vi "Read.vi"(8 "error in (no error)":errorcluster) -> (0 "error out":errorcluster)   [LabVIEW 2018, in "text_file.lvlib"]
doc: "Reads all text (all contents) of file."
uses:
  text_file.lvlib
  private_data (library_variable).vi
panel:
  out "Text read from file (contents of file)":string
  # "Development\ncontrols/indicators useful for development and testing, but which are not outputs of the VI"
  # "Input\nInputs to the VI"
  # "Output\nOutputs of the VI"
  # "Description\n\nBlank VI with error handling case. \n\nSummarize the use of this VI in this space."
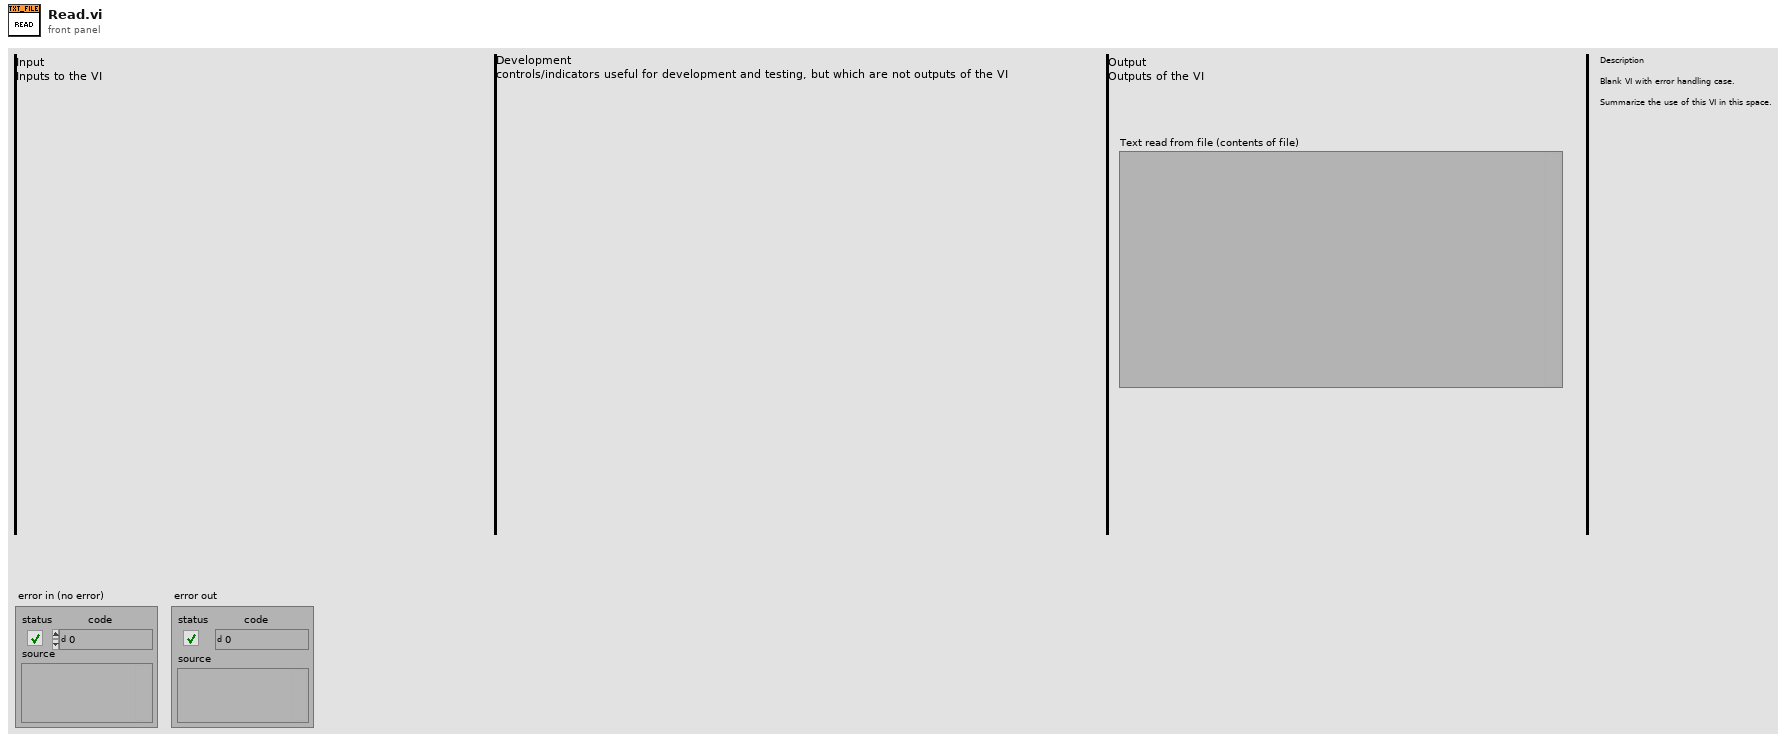
[diagram p1: front panel]
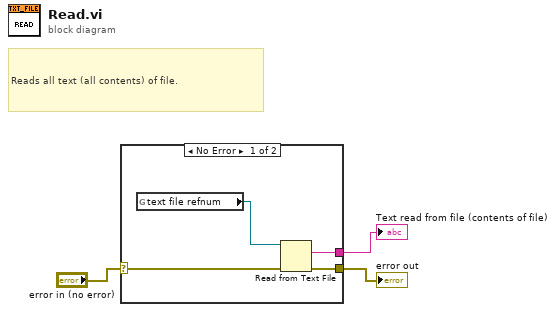
[diagram p0: block diagram]
diagram:
  # "Reads all text (all contents) of file."
  n1 = case shown="No Error" "error in (no error)" {
    selector: "error in (no error)" -> [w7 w8]
    tunnel: [w6 w8] -> w2
    tunnel: [w4 _] -> w1
    frame No Error {
      n2 = global read "private_data (library_variable).vi" "text file refnum"() -> (w5:refnum<file>)
      n3 = Read from Text File(file (use dialog)=w5, error in=w7) -> (text=w4:string, error out=w6:errorcluster)  [unwired: 2 in, 2 out]
    }
    frame Error {
    }
  }
  "error out" <- w2
  "Text read from file (contents of file)" <- w1
